vi "ExSubStreamCol.vi"(2 "error in (no error)":errorcluster, 3 "Handle Cluster":T1) -> (0 "error out":errorcluster, 1 "Handle Cluster":T1)   [LabVIEW 2010]
panel:
  # "ExSubStreamCol:\nThis is a sub VI that collects stream mode from \nthe camera system. This assumes camera has \nbeen setup and initialized and that the start \ncamera is done."
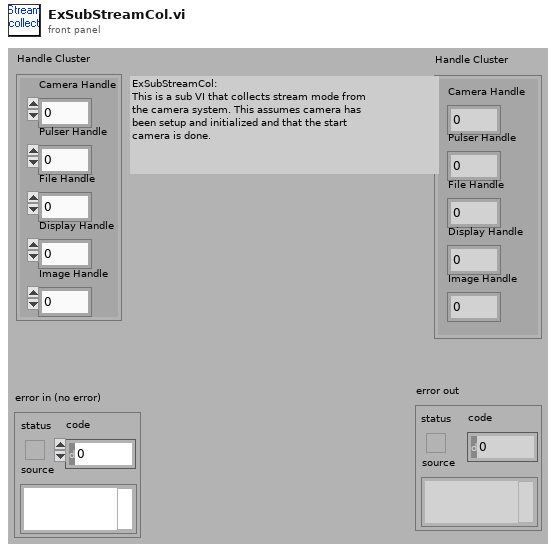
[diagram p1: front panel]
types:
  T1 = cluster{"Camera Handle":u32, "Pulser Handle":u32, "File Handle":u32, "Display Handle":u32, "Image Handle":u32}
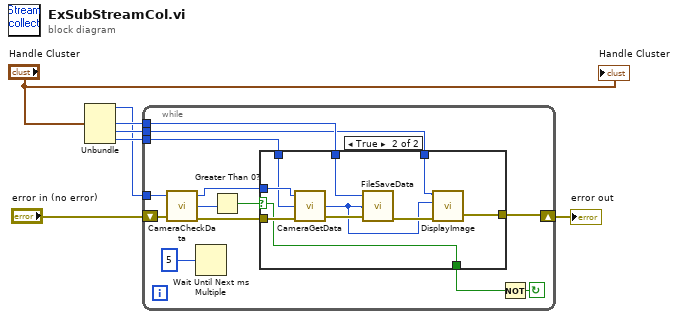
[diagram p0: block diagram]
diagram:
  n1 = Unbundle("Handle Cluster") -> ("Camera Handle"=w3:u32, "File Handle"=w5:u32, "Display Handle"=w4:u32, "Image Handle"=w6:u32)  [unwired: 1 out]
  n2 = while {
    tunnel: w6 -> [w16]
    tunnel: w5 -> [w15]
    tunnel: w4 -> [w14]
    tunnel: w3 -> [w13]
    shift-right: [w11] -> w1
    shift-left: "error in (no error)" -> [w12]
    stop <- w9 continue-if-true
    n3 = call <userlib>:"CameraCheckData.vi"("Camera Handle"=w13, "error in"=w12) -> ("Camera Handle"=w19:u32, "Number Of Frames Available"=w20:i32, "error out"=w18:errorcluster)
    n4 = Wait Until Next ms Multiple(millisecond multiple=u32 5) -> ()  [unwired: 1 out]
    n5 = Greater Than 0?(x=w20) -> (x > 0?=w10:bool)
    n6 = case shown="True" w10 {
      selector: w10 -> [w21 w23]
      tunnel: w19 -> [_ w32]
      tunnel: [w22 w29] -> w11
      tunnel: w18 -> [w22 w28]
      tunnel: w16 -> [_ w27]
      tunnel: w15 -> [_ w26]
      tunnel: w14 -> [_ w24]
      tunnel: [w21 w23] -> w8
      frame False {
      }
      frame True {
        n7 = call <userlib>:"CameraGetData.vi"("error in"=w28, "Data Handle"=w27, "Camera Handle"=w32) -> ("error out"=w31:errorcluster, "Data Handle"=w25:u32)  [unwired: 1 out]
        n8 = call <userlib>:"FileSaveData.vi"("error in"=w31, "Image Handle"=w25, "File Handle"=w26) -> ("error out"=w30:errorcluster)  [unwired: 1 out]
        n9 = call <userlib>:"DisplayImage.vi"("error in"=w30, "Image Handle"=w25, "Display Handle"=w24) -> ("error out"=w29:errorcluster)  [unwired: 1 in, 1 out]
      }
    }
    n10 = Not(x=w8) -> (.not. x?=w9:bool)
  }
  "error out" <- w1
  "Handle Cluster" <- "Handle Cluster"
